vi "CANOpen_SDO Dynamic -Create Channels.vi"(8 "error in (no error)":errorcluster, 11 "Section Ptr":T1 format="%.0x") -> (0 "error out":errorcluster)   [LabVIEW 2013, in "CANOpen Addon Custom Device.lvlib"]
uses:
  CANOpen Addon Custom Device.lvlib
  <vilib>/NI Veristand/Custom Device API/Custom Device Item Ref.ctl
  <vilib>/NI Veristand/Custom Device API/Custom Device Channel.ctl
  <vilib>/NI Veristand/Custom Device API/Custom Device Channel Type.ctl
  Shared Code/CANOpen Addon GUID Lookup Global.vi
  <vilib>/NI Veristand/Custom Device API/Custom Device API.lvlib
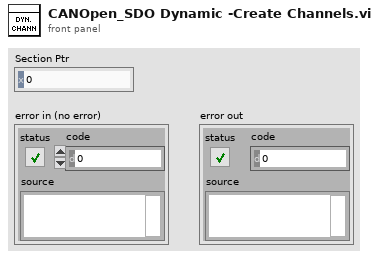
[diagram p1: front panel]
types:
  T1 = typedef "Custom Device API.lvlib/Custom Device Item Ref.ctl" = u64
  T2 = typedef "Custom Device API.lvlib/Custom Device Channel.ctl" = cluster{"Type":T3, "Units":string, "Default Value":dbl, "Faultable":bool, "Scalable":bool}
  T3 = typedef "Custom Device API.lvlib/Custom Device Channel Type.ctl" = enum16{"Input", "Output"}
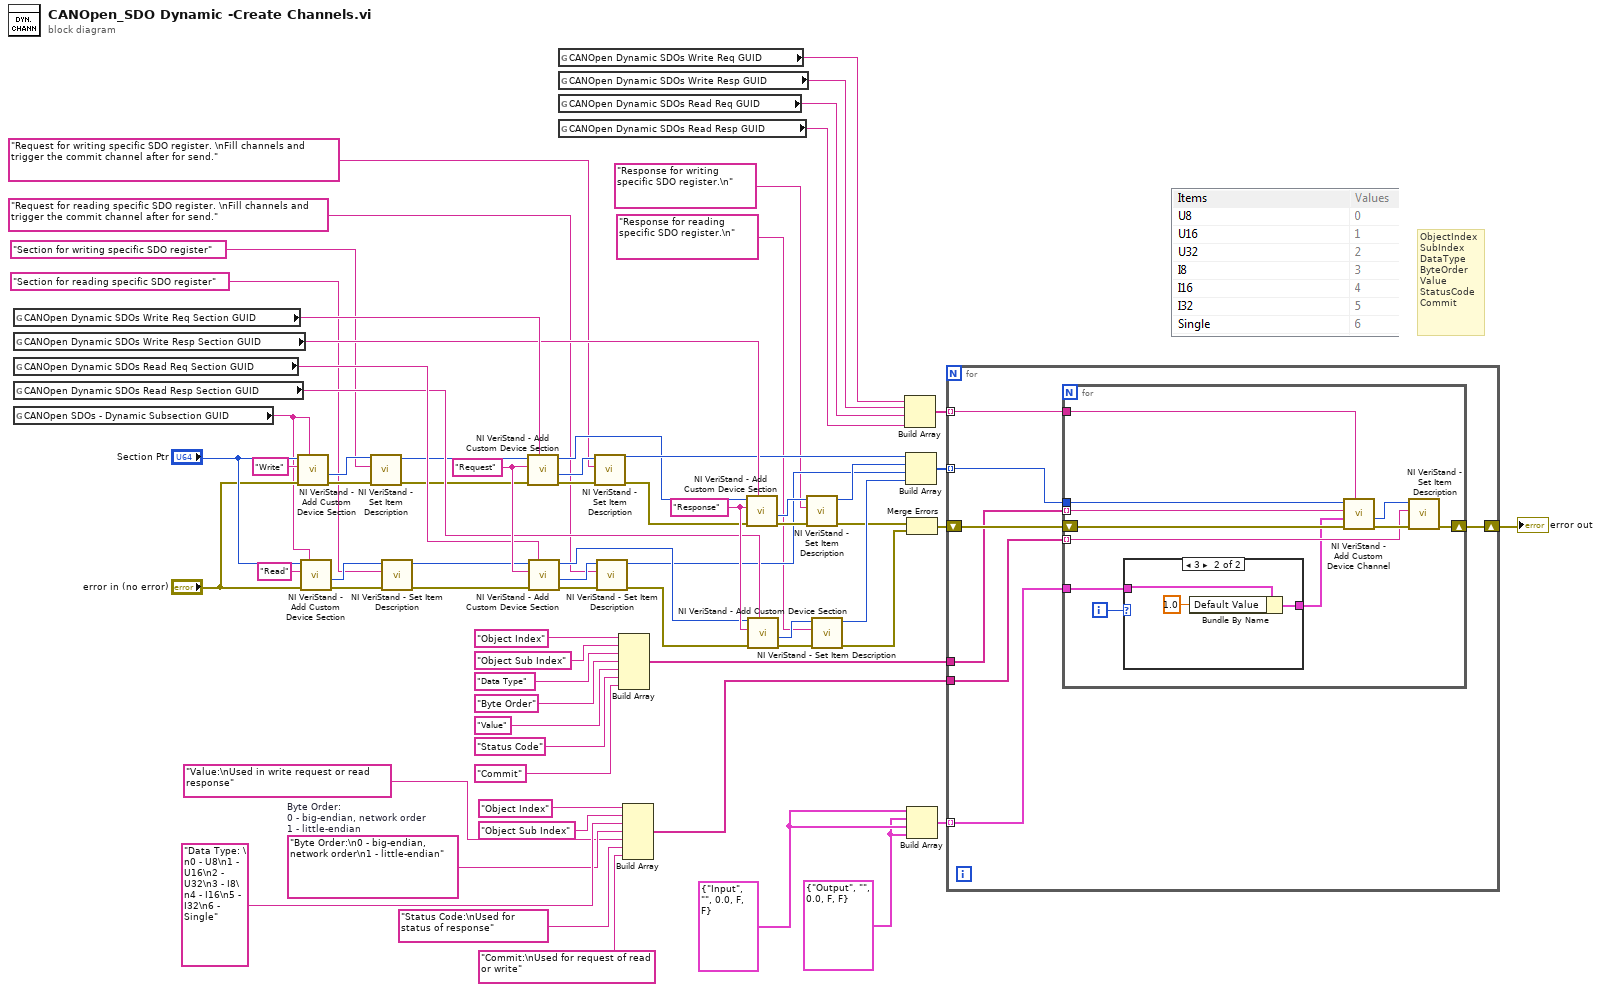
[diagram p0: block diagram]
diagram:
  w42 = T2 {"Type"=enum."Output", "Units"="", "Default Value"=0.0, "Faultable"=FALSE, "Scalable"=FALSE} ("Channel")
  w43 = T2 {"Type"=enum."Input", "Units"="", "Default Value"=0.0, "Faultable"=FALSE, "Scalable"=FALSE} ("Channel")
  w54 = "Byte Order:\n0 - big-endian, network order\n1 - little-endian"  # Byte Order: 0 - big-endian, network order 1 - little-endian
  w38 = "Response" ("Section Name")
  w39 = "Request" ("Section Name")
  # "ObjectIndex\nSubIndex\nDataType\nByteOrder\nValue\nStatusCode\nCommit"
  n1 = global read "CANOpen Addon GUID Lookup Global.vi" "CANOpen Dynamic SDOs Write Req Section GUID"() -> (w37:string)
  n2 = global read "CANOpen Addon GUID Lookup Global.vi" "CANOpen Dynamic SDOs Write Resp Section GUID"() -> (w36:string)
  n3 = global read "CANOpen Addon GUID Lookup Global.vi" "CANOpen Dynamic SDOs Read Req Section GUID"() -> (w35:string)
  n4 = global read "CANOpen Addon GUID Lookup Global.vi" "CANOpen Dynamic SDOs Read Resp Section GUID"() -> (w34:string)
  n5 = global read "CANOpen Addon GUID Lookup Global.vi" "CANOpen SDOs - Dynamic Subsection GUID"() -> (w33:string)
  n6 = call <vilib>:"NI VeriStand - Add Custom Device Section.vi"("GUID (Default Section)"=w33, "error in (no error)"="error in (no error)", "Section Name"="Write", "Parent Ref in"="Section Ptr") -> ("error out"=w24:errorcluster, "Section Ptr"=w22:T1)  [unwired: 4 in, 2 out]
  n7 = call <vilib>:"NI VeriStand - Add Custom Device Section.vi"("GUID (Default Section)"=w33, "error in (no error)"="error in (no error)", "Section Name"="Read", "Parent Ref in"="Section Ptr") -> ("error out"=w20:errorcluster, "Section Ptr"=w17:T1)  [unwired: 4 in, 2 out]
  n8 = call <vilib>:"NI VeriStand - Set Item Description.vi"("error in (no error)"=w24, "Description"="Section for writing specific SDO register", "Item Ref in"=w22) -> ("error out"=w23:errorcluster, "Item Ref out"=w21:T1)  [unwired: 6 in, 1 out]
  n9 = call <vilib>:"NI VeriStand - Set Item Description.vi"("error in (no error)"=w20, "Description"="Section for reading specific SDO register", "Item Ref in"=w17) -> ("error out"=w19:errorcluster, "Item Ref out"=w18:T1)  [unwired: 6 in, 1 out]
  n10 = call <vilib>:"NI VeriStand - Add Custom Device Section.vi"("GUID (Default Section)"=w37, "error in (no error)"=w23, "Section Name"=w39, "Parent Ref in"=w21) -> ("error out"=w16:errorcluster, "Section Ptr"=w14:T1, "Parent Ref out"=w12:T1)  [unwired: 4 in, 1 out]
  n11 = call <vilib>:"NI VeriStand - Add Custom Device Section.vi"("GUID (Default Section)"=w35, "error in (no error)"=w19, "Section Name"=w39, "Parent Ref in"=w18) -> ("error out"=w10:errorcluster, "Section Ptr"=w7:T1, "Parent Ref out"=w11:T1)  [unwired: 4 in, 1 out]
  n12 = global read "CANOpen Addon GUID Lookup Global.vi" "CANOpen Dynamic SDOs Write Req GUID"() -> (w48:string)
  n13 = global read "CANOpen Addon GUID Lookup Global.vi" "CANOpen Dynamic SDOs Write Resp GUID"() -> (w47:string)
  n14 = global read "CANOpen Addon GUID Lookup Global.vi" "CANOpen Dynamic SDOs Read Req GUID"() -> (w46:string)
  n15 = global read "CANOpen Addon GUID Lookup Global.vi" "CANOpen Dynamic SDOs Read Resp GUID"() -> (w45:string)
  n16 = call <vilib>:"NI VeriStand - Set Item Description.vi"("error in (no error)"=w16, "Description"="Request for writing specific SDO register. \nFill channels and trigger the commit channel after for send.", "Item Ref in"=w14) -> ("error out"=w15:errorcluster, "Item Ref out"=w13:T1)  [unwired: 6 in, 1 out]
  n17 = call <vilib>:"NI VeriStand - Set Item Description.vi"("error in (no error)"=w10, "Description"="Request for reading specific SDO register. \nFill channels and trigger the commit channel after for send.", "Item Ref in"=w7) -> ("error out"=w9:errorcluster, "Item Ref out"=w8:T1)  [unwired: 6 in, 1 out]
  n18 = Build Array("Object Index", "Object Sub Index", "Data Type", "Byte Order", "Value", "Status Code", "Commit") -> (w50:string[])
  n19 = Build Array("Object Index", "Object Sub Index", "Data Type: \n0 - U8\n1 - U16\n2 - U32\n3 - I8\n4 - I16\n5 - I32\n6 - Single", w54, "Value:\nUsed in write request or read response", "Status Code:\nUsed for status of response", "Commit:\nUsed for request of read or write") -> (w40:string[])
  n20 = call <vilib>:"NI VeriStand - Add Custom Device Section.vi"("GUID (Default Section)"=w36, "error in (no error)"=w15, "Section Name"=w38, "Parent Ref in"=w12) -> ("error out"=w28:errorcluster, "Section Ptr"=w25:T1)  [unwired: 4 in, 2 out]
  n21 = call <vilib>:"NI VeriStand - Add Custom Device Section.vi"("GUID (Default Section)"=w34, "error in (no error)"=w9, "Section Name"=w38, "Parent Ref in"=w11) -> ("error out"=w32:errorcluster, "Section Ptr"=w29:T1)  [unwired: 4 in, 2 out]
  n22 = call <vilib>:"NI VeriStand - Set Item Description.vi"("error in (no error)"=w28, "Description"="Response for writing specific SDO register.\n", "Item Ref in"=w25) -> ("error out"=w27:errorcluster, "Item Ref out"=w26:T1)  [unwired: 6 in, 1 out]
  n23 = call <vilib>:"NI VeriStand - Set Item Description.vi"("error in (no error)"=w32, "Description"="Response for reading specific SDO register.\n", "Item Ref in"=w29) -> ("error out"=w31:errorcluster, "Item Ref out"=w30:T1)  [unwired: 6 in, 1 out]
  n24 = Build Array(w48, w47, w46, w45) -> (w44:string[])
  n25 = Build Array(w13, w26, w8, w30) -> (w65:T1[])
  n26 = Merge Errors(w27, w31) -> (w68:errorcluster)
  n27 = Build Array(w43, w42, w43, w42) -> (w41:T2[])
  n28 = for {
    shift-right: [w76] -> w49
    shift-left: w68 -> [w77]
    tunnel: w65 -> [w74] mode=indexing
    tunnel: w50 -> [w75]
    tunnel: w44 -> [w73] mode=indexing
    tunnel: w41 -> [w72] mode=indexing
    tunnel: w40 -> [w71]
    n29 = for {
      shift-right: [w83] -> w76
      shift-left: w77 -> [w88]
      tunnel: w75 -> [w87] mode=indexing
      tunnel: w74 -> [w86]
      tunnel: w73 -> [w82]
      tunnel: w72 -> [w79]
      tunnel: w71 -> [w81] mode=indexing
      i -> [w80]
      n30 = case shown="3" w80 {
        tunnel: w79 -> [w89 w92]
        tunnel: [w89 w91] -> w78
        frame 0, Default {
        }
        frame 3 {
          n31 = Bundle By Name(cluster=w92, "Default Value"=1.0) -> (w91:T2)
        }
      }
      n32 = call <vilib>:"NI VeriStand - Add Custom Device Channel.vi"("GUID (Default Channel)"=w82, "error in (no error)"=w88, "Channel"=w78, "Channel Name"=w87, "Parent Ref in"=w86) -> ("error out"=w84:errorcluster, "Channel Ref"=w85:T1)  [unwired: 3 in, 2 out]
      n33 = call <vilib>:"NI VeriStand - Set Item Description.vi"("error in (no error)"=w84, "Description"=w81, "Item Ref in"=w85) -> ("error out"=w83:errorcluster)  [unwired: 6 in, 2 out]
    }
  }
  "error out" <- w49
